vi "mod_FM CE Modulation.vi"(0 "x":dbl[](array[numeric]), 1 "carrier phase [rad]":dbl, 5 "fs":dbl, 9 "kf":dbl, 12 "reset?":bool) -> (4 "FM CE":cdb[](array[numeric]))   [LabVIEW 2020, in "niAMT.lvlib"]
uses:
  <vilib>/addons/Modulation/niAMT.lvlib
  nilvamt.dll
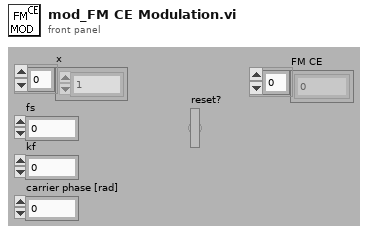
[diagram p1: front panel]
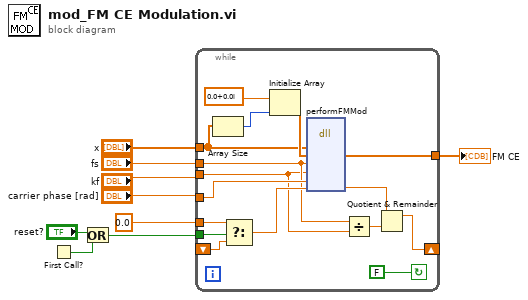
[diagram p0: block diagram]
diagram:
  n1 = First Call?() -> (First Call?: T/F=w5:bool)
  n2 = Or(x="reset?", y=w5) -> (x .or. y?=w3:bool)
  n3 = while {
    tunnel: "x" -> [w14]
    tunnel: "fs" -> [w18]
    tunnel: "kf" -> [w17]
    tunnel: "carrier phase [rad]" -> [w25]
    shift-right: [w15] -> _
    shift-left: _ -> [w23]
    tunnel: w3 -> [w10]
    tunnel: 0.0 ("Initial Y value") -> [w21]
    tunnel: [w12] -> w1
    stop <- FALSE continue-if-true
    n4 = Array Size(array=w14) -> (size(s)=w13:i32)
    n5 = Select(t=w21, s=w10, f=w23) -> (s? t:f=w22:dbl)
    n6 = Initialize Array(cdb 0.0+0.0i ("element"), w13) -> (w19:cdb[])
    n7 = dll-call lib="nilvamt.*" fn="performFMMod" ("FM_mod.dll:performFM_mod2")("DataIN"=w14, "DataOut"=w19, "SamplFreq"=w18, "FreqDev"=w17, "CarrFreq"=w25, "initialYvalue"=w22) -> ("DataOut"=w12:cdb[], "initialYvalue"=w11:dbl)  [unwired: 7 in, 3 out]
    n8 = Divide(x=w18, y=w17) -> (x/y=w16:dbl)
    n9 = Quotient & Remainder(x=w11, y=w16) -> (x-y*floor(x/y)=w15:dbl)  [unwired: 1 out]
  }
  "FM CE" <- w1
